vi "ScanAction.vi"(8 "error in (no error)":errorcluster caption="entrée d'erreur (pas d'erreur)", 9 "IndicePoint":i32, 10 "Dir":bool, 11 "Tools In":refnum<class "AttoAMC.lvclass"> caption="DNL_LabVIEW Object in") -> (0 "error out":errorcluster caption="sortie d'erreur", 2 "ScanParsOut":dbl[](array[numeric]), 3 "Tools Out":refnum<class "AttoAMC.lvclass"> caption="DNL_LabVIEW Object out")   [LabVIEW 2019, in "AttoAMC.lvclass"]
uses:
  AttoAMC.lvclass
  C:/Programmes Labview/LabScanV1A/DevicesClass/BaseDevice/BaseDevice.lvclass
  AttoAMC.lvclass/AttoAMC.ctl
  ScanActionStates.ctl
  <userlib>/GenProg/WritebyWeakRefNum.vi
  <vilib>/Utility/error.llb/Error Cluster From Error Code.vi
  <vilib>/ErrorRing/Error Ring.xnode
panel:
  in  "Reactivate":bool
  out "axis":u8
  out "Bkwd":bool
  out "Fwd":bool
  out "Trgt Rng(nm)":dbl
  in  "CtrlLpReact":u32
  out "PosDiff(nm)":dbl
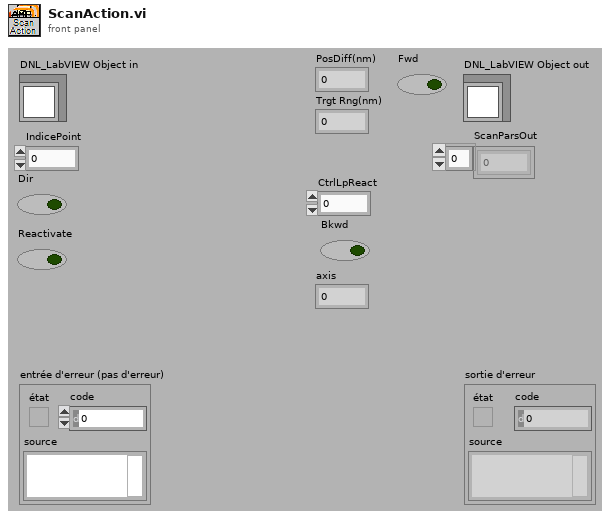
[diagram p1: front panel]
types:
  T1 = typedef "ScanActionStates.ctl" = enum16{"ReadPosDiff", "SetTarget", "WaitMoveDone", "MoveDone", "Timeout", "Ctrl_Loop_React", "Limit_check", "Error"}
  T2 = typedef "AttoAMC.lvclass/AttoAMC_Func.ctl" = enum16{"Position (um)"}
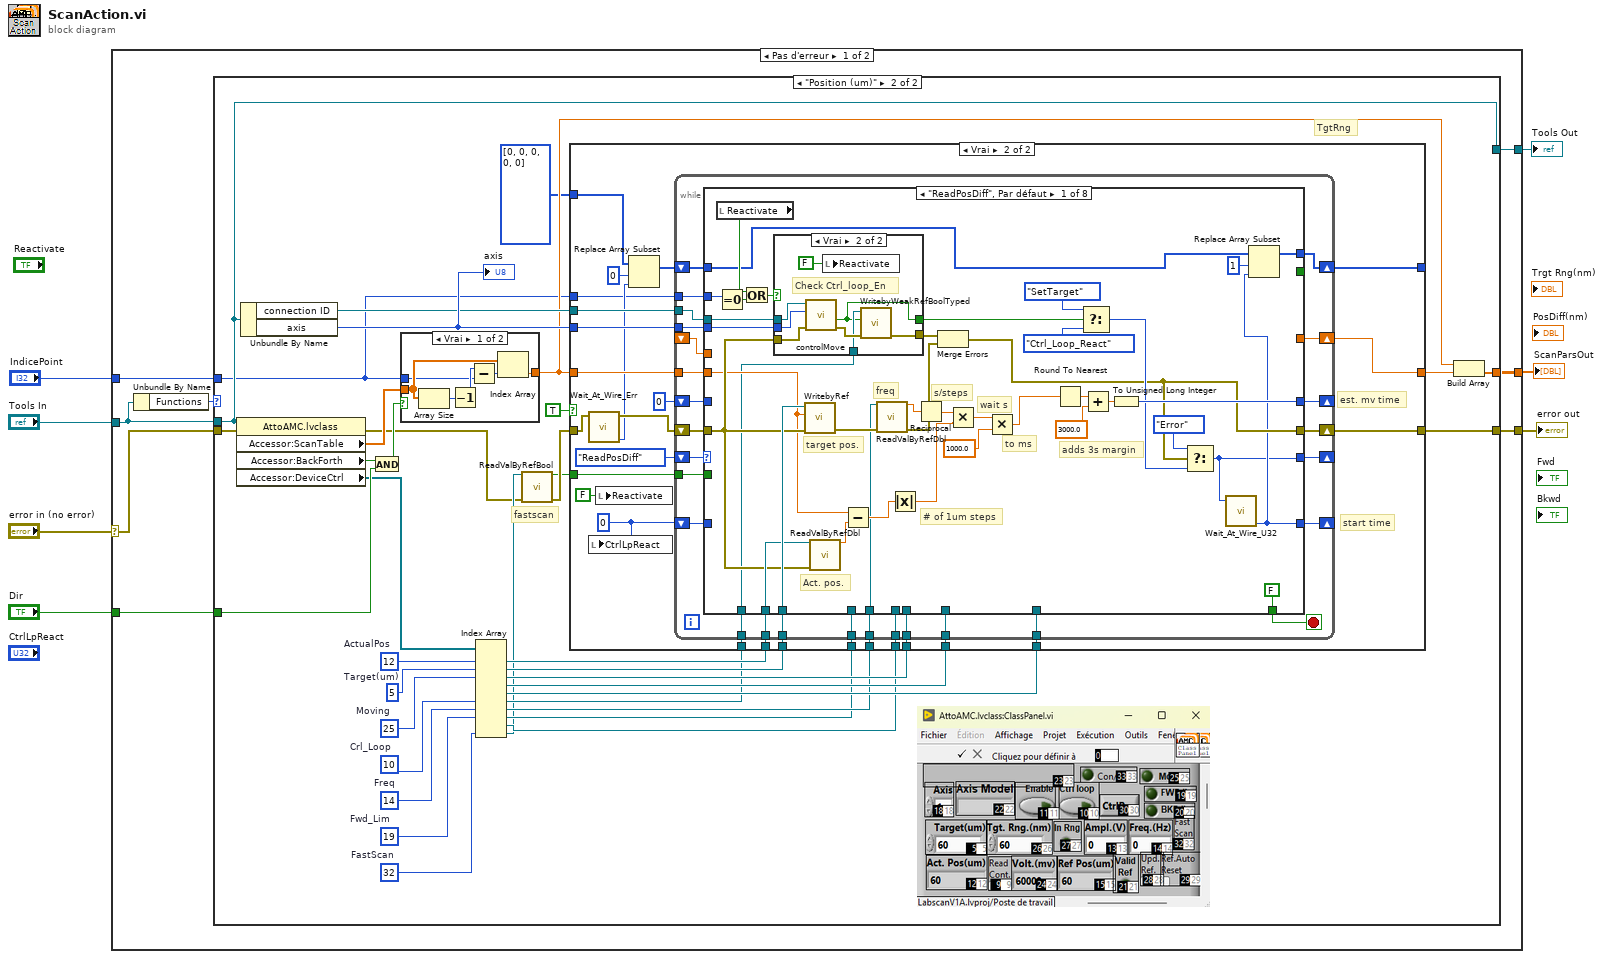
[diagram p0: block diagram]
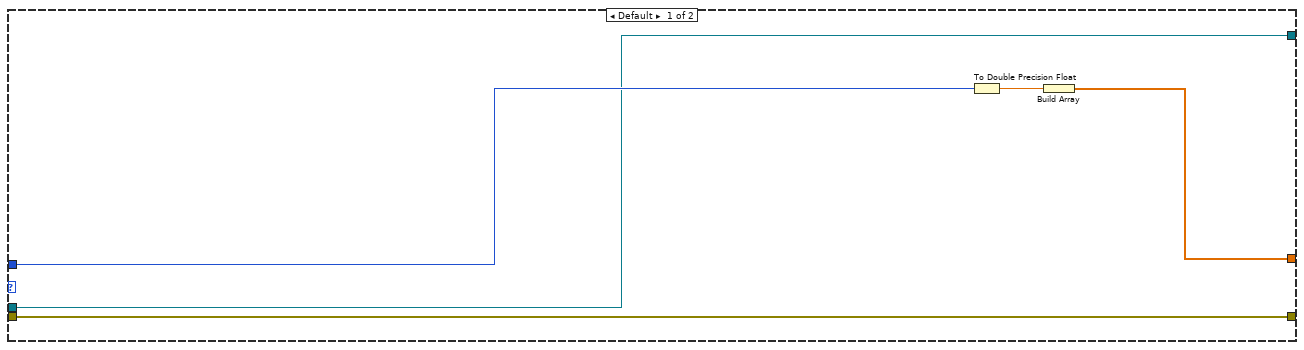
[diagram p2: hidden frame]
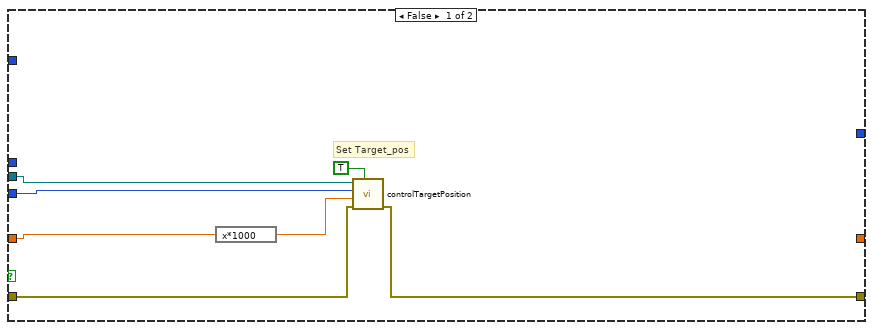
[diagram p3: hidden frame]
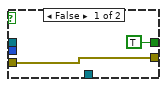
[diagram p4: hidden frame]
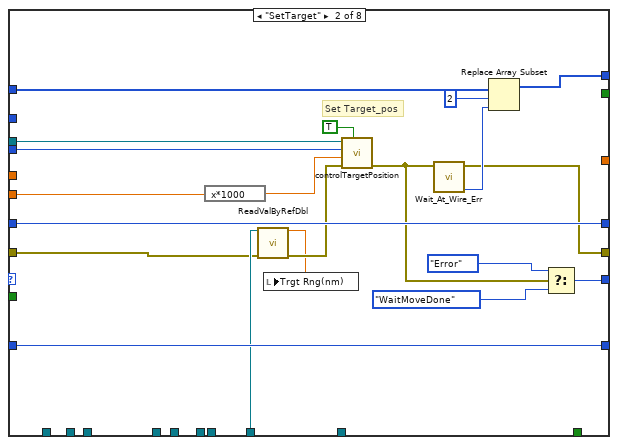
[diagram p5: hidden frame]
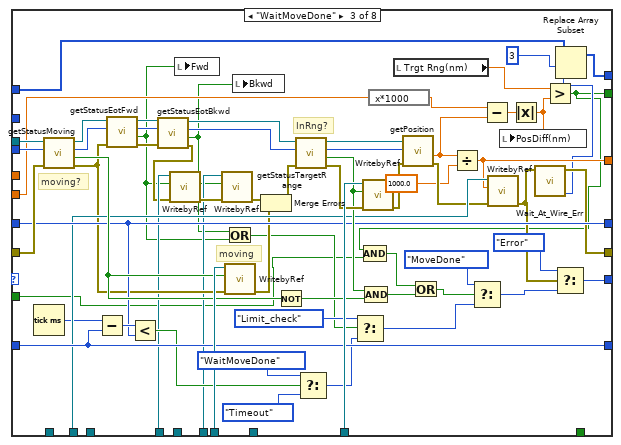
[diagram p6: hidden frame]
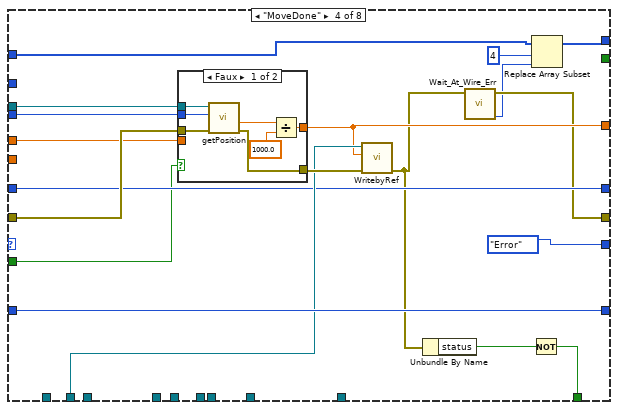
[diagram p7: hidden frame]
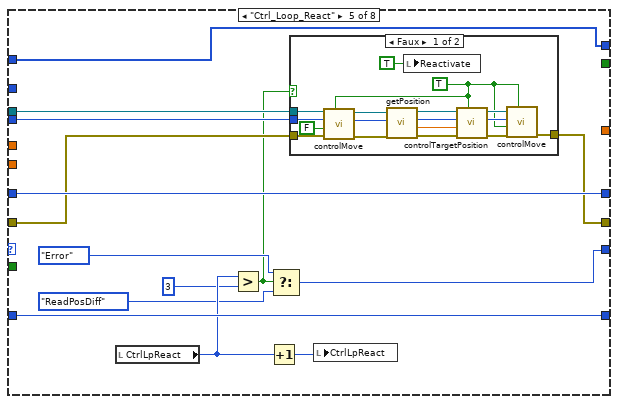
[diagram p9: hidden frame]
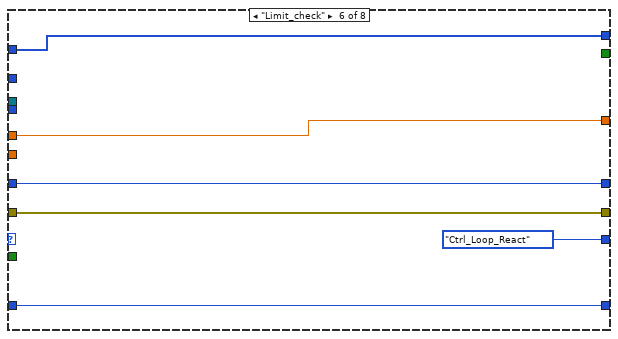
[diagram p11: hidden frame]
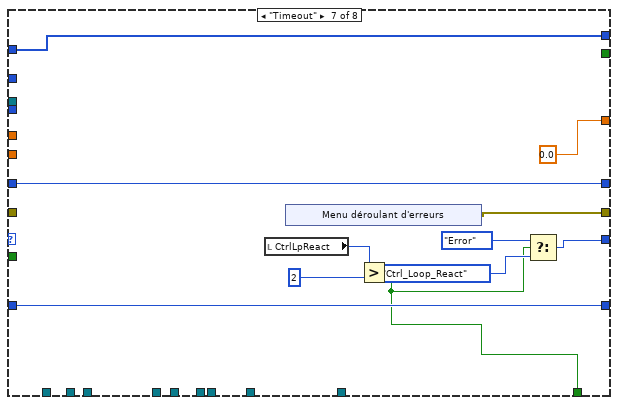
[diagram p12: hidden frame]
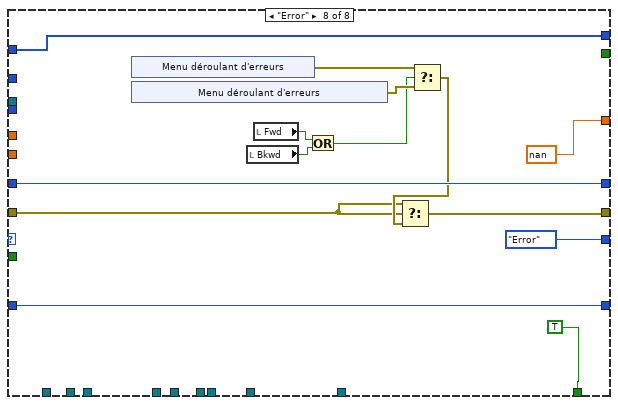
[diagram p13: hidden frame]
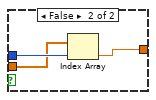
[diagram p14: hidden frame]
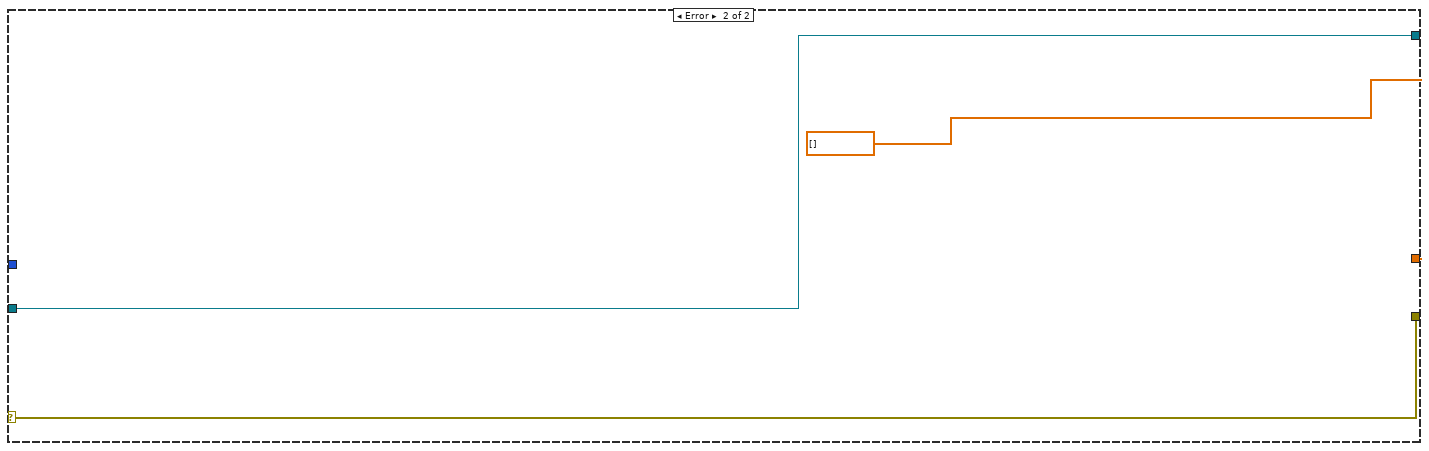
[diagram p15: hidden frame]
diagram:
  n1 = case shown="Pas d'erreur" "error in (no error)" {
    selector: "error in (no error)" -> [w12 w369]
    tunnel: "Tools In" -> [w13 w368]
    tunnel: [w11 dbl[] []] -> w2
    tunnel: [w10 w369] -> w5
    tunnel: [w9 w368] -> w4
    tunnel: "IndicePoint" -> [w14 _]
    tunnel: "Dir" -> [w8 _]
    frame No Error {
      n2 = Unbundle By Name(w13) -> ("Functions"=w15:T2)
      n3 = case shown="\"Position (um)\"" w15 {
        tunnel: [w16 w56] -> w11
        tunnel: w14 -> [w20 w21]
        tunnel: [w18 w55] -> w9
        tunnel: w13 -> [w18 w55]
        tunnel: w12 -> [w17 w54]
        tunnel: [w17 w42] -> w10
        tunnel: w8 -> [_ w50]
        frame Default {
          n4 = To Double Precision Float(number=w20) -> (double precision float=w19:dbl)
          n5 = Build Array(w19) -> (w16:dbl[])
        }
        frame "Position (um)" {
          w26 = 32  # FastScan
          w32 = 19  # Fwd_Lim
          w34 = 14  # Freq
          w36 = 10  # Crl_Loop
          w44 = 5  # Target(um)
          w47 = 25  # Moving
          w48 = 12  # ActualPos
          # "fastscan"
          # "TgtRng"
          n6 = property class="AttoAMC.lvclass"(reference=w55, error in=w54) -> (error out=w24:errorcluster, "Accessor:ScanTable"=w53:dbl[], "Accessor:BackForth"=w52:bool, "Accessor:DeviceCtrl"=w49:refnum<vi>[])  [unwired: 1 out]
          n7 = Unbundle By Name(w55) -> ("connection ID"=w40:refnum<k5>, "axis"=w41:u8)
          "axis" <- w41
          n8 = And(x=w52, y=w50) -> (x .and. y?=w51:bool)
          n9 = case shown="Vrai" w51 {
            tunnel: w21 -> [w358 w366]
            tunnel: [w363 w364] -> w29
            tunnel: w53 -> [w362 w365]
            frame True {
              n10 = Array Size(array=w362) -> (size(s)=w361:i32)
              n11 = Decrement(x=w361) -> (x-1=w359:i32)
              n12 = Subtract(x=w359, y=w358) -> (x-y=w360:i32)
              n13 = Index Array(array=w362, index=w360) -> (element=w363:dbl)
            }
            frame False {
              n14 = Index Array(array=w365, index=w366) -> (element=w364:dbl)
            }
          }
          n15 = Index Array(array=w49, index #1=w48, index #2=w44, index #3=w47, index #6=w36, index #7=w34, index #8=w32, index #10=w26) -> (element #1=w39:refnum<vi>, element #2=w45:refnum<vi>, element #3=w46:refnum<vi>, element #4=w37:refnum<vi>, element #5=w38:refnum<vi>, element #6=w35:refnum<vi>, element #7=w33:refnum<vi>, element #8=w31:refnum<vi>, element #9=w30:refnum<vi>, element #10=w25:refnum<vi>)  [unwired: 3 in]
          n16 = call <userlib>:"ReadValByRefBool.vi"("Control Ref"=w25, "error in"=w24) -> ("Valeur"=w22:bool, "error out"=w23:errorcluster)  [unwired: 12 in]
          n17 = case shown="Vrai" TRUE {
            tunnel: w46 -> [_ w90]
            tunnel: w45 -> [_ w89]
            tunnel: [_ w88] -> w43
            tunnel: [w57 w87] -> w42
            tunnel: w41 -> [w60 w86]
            tunnel: w40 -> [w61 w85]
            tunnel: w23 -> [w58 w73]
            tunnel: w39 -> [_ w84]
            tunnel: w38 -> [_ w81]
            tunnel: w37 -> [_ w80]
            tunnel: w35 -> [_ w79]
            tunnel: w33 -> [_ w78]
            tunnel: w31 -> [_ w77]
            tunnel: w30 -> [_ w76]
            tunnel: w29 -> [w59 w75]
            tunnel: u32[] [0, 0, 0, 0, 0] ("Clock(ms)") -> [_ w70]
            tunnel: [_ w67] -> _
            tunnel: w22 -> [_ w66]
            tunnel: w21 -> [_ w65]
            frame False {
              # "Set Target_pos"
              n18 = expression code="x*1000"(w59) -> (w62:dbl)
              n19 = call <userlib>:"controlTargetPosition.vi"("Set"=TRUE, "error in"=w58, "Target Position in"=w62, "axis in"=w60, "connection ID"=w61) -> ("error out"=w57:errorcluster)  [unwired: 3 in, 3 out]
            }
            frame True {
              w74 = u32 0 ("millisecond timer value")
              # "est. mv time"
              # "start time"
              n20 = call <userlib>:"Wait_At_Wire_Err.vi"("error in (no error)"=w73) -> ("Clock(ms)"=w68:u32, "error out"=w72:errorcluster)  [unwired: 8 in, 1 out]
              n21 = local write "CtrlLpReact"(w74) -> ()
              n22 = local write "Reactivate"(FALSE ("Reactivate")) -> ()
              n23 = Replace Array Subset(array=w70, new element=w68, index=0 ("indice")) -> (w71:u32[])
              n24 = while {
                tunnel: w90 -> [w117]
                tunnel: w89 -> [w116]
                tunnel: w81 -> [w114]
                tunnel: w86 -> [w112]
                tunnel: w85 -> [w111]
                tunnel: w84 -> [w109]
                shift-right: [w113] -> w87
                shift-left: w72 -> [w110]
                shift-right: [w106] -> _
                shift-left: w74 -> [w103]
                shift-right: [w105] -> _
                shift-left: ScanActionStates."ReadPosDiff" -> [w107]
                shift-right: [w102] -> _
                shift-left: u32 0 -> [w101]
                tunnel: w80 -> [w100]
                tunnel: w79 -> [w99]
                tunnel: w78 -> [w98]
                tunnel: w77 -> [w97]
                tunnel: w76 -> [w96]
                tunnel: w75 -> [w108]
                shift-right: [w95] -> w67
                shift-left: w71 -> [w94]
                tunnel: w66 -> [w93]
                tunnel: w65 -> [w92]
                shift-right: [w115] -> w88
                shift-left: _ -> [w91]
                stop <- w104 stop-if-true
                n25 = case shown="\"ReadPosDiff\", Par défaut" w107 {
                  tunnel: w117 -> [_ _ w251 _ _ _ _ _]
                  tunnel: w116 -> [w156 _ _ _ _ _ _ _]
                  tunnel: [_ _ w205 w264 _ w312 0.0 ("ScanParamIn") nan ("ScanParamIn")] -> w115
                  tunnel: w114 -> [_ _ w250 _ _ _ _ _]
                  tunnel: [w135 w167 w193 w258 w282 w315 w325 w335] -> w113
                  tunnel: w112 -> [w143 w177 w246 w266 w290 _ _ _]
                  tunnel: w111 -> [w144 w178 w247 w267 w291 _ _ _]
                  tunnel: w110 -> [w142 w179 w245 w265 w289 w315 _ w336]
                  tunnel: w109 -> [w152 _ w231 w268 _ _ _ _]
                  tunnel: w108 -> [w134 w175 w204 _ _ _ _ _]
                  tunnel: [w122 w183 w244 w269 w292 w316 w328 w345] -> w106
                  tunnel: [w121 w184 w235 ScanActionStates."Error" w283 ScanActionStates."Ctrl_Loop_React" w319 ScanActionStates."Error"] -> w105
                  tunnel: [FALSE _ _ w261 _ _ w320 TRUE] -> w104
                  tunnel: w103 -> [_ w183 w244 w269 w292 w316 w328 w345]
                  tunnel: [w148 w182 w241 w263 w293 w317 w327 w344] -> w102
                  tunnel: w101 -> [_ w182 w241 w263 w293 w317 w327 w344]
                  tunnel: w100 -> [_ w180 _ _ _ _ _ _]
                  tunnel: [_ _ w188 _ _ _ _ _] -> _
                  tunnel: w99 -> [w125 _ _ _ _ _ _ _]
                  tunnel: w98 -> [w146 _ _ _ _ _ _ _]
                  tunnel: w97 -> [_ _ w219 _ _ _ _ _]
                  tunnel: w96 -> [_ _ w218 _ _ _ _ _]
                  tunnel: [w127 w170 w197 w254 w280 w313 w318 w334] -> w95
                  tunnel: w94 -> [w118 w171 w196 w255 w280 w313 w318 w334]
                  tunnel: w93 -> [_ _ w189 w252 _ _ _ _]
                  tunnel: w92 -> [w124 _ _ _ _ _ _ _]
                  tunnel: w91 -> [_ _ _ w253 _ w312 _ _]
                  frame "ReadPosDiff", Default {
                    # "adds 3s margin"
                    # "to ms"
                    # "freq"
                    # "s/steps"
                    # "wait s"
                    # "# of 1um steps"
                    # "Act. pos."
                    # "target pos."
                    n26 = local read "Reactivate"() -> (w119:bool)
                    n27 = Equal To 0?(x=w124) -> (x = 0?=w123:bool)
                    n28 = Or(x=w119, y=w123) -> (x .or. y?=w120:bool)
                    n29 = case shown="Vrai" w120 {
                      tunnel: w144 -> [_ w166]
                      tunnel: w143 -> [_ w165]
                      tunnel: w142 -> [w158 w160]
                      tunnel: [w158 w163] -> w140
                      tunnel: [TRUE ("controll move out") w161] -> w136
                      tunnel: w125 -> [_ w162]
                      frame False {
                      }
                      frame True {
                        # "Check Ctrl_loop_En"
                        n30 = call <userlib>:"controlMove.vi"("error in"=w160, "axis in"=w165, "connection ID"=w166) -> ("error out"=w164:errorcluster, "controll move out"=w161:bool)  [unwired: 5 in, 2 out]
                        n31 = local write "Reactivate"(FALSE ("Reactivate")) -> ()
                        n32 = call <userlib>:"WritebyWeakRefBoolTyped.vi"("error in"=w164, "Valeur"=w161, "Control Ref"=w162) -> ("error out"=w163:errorcluster)  [unwired: 8 in]
                      }
                    }
                    n33 = call-poly <userlib>:"WritebyRef.vi"("error in"=w142, "Valeur"=w134, "Control Ref"=w156) -> ("error out"=w147:errorcluster)  [unwired: 8 in]
                    n34 = call <userlib>:"ReadValByRefDbl.vi"("Control Ref"=w152, "error in"=w142) -> ("Valeur"=w155:dbl)  [unwired: 12 in, 1 out]
                    n35 = Subtract(x=w134, y=w155) -> (x-y=w154:dbl)
                    n36 = call <userlib>:"ReadValByRefDbl.vi"("Control Ref"=w146, "error in"=w147) -> ("Valeur"=w145:dbl, "error out"=w141:errorcluster)  [unwired: 12 in]
                    n37 = Absolute Value(x=w154) -> (abs(x)=w131:dbl)
                    n38 = Reciprocal(x=w145) -> (1/x=w153:dbl)
                    n39 = Merge Errors(w140, w141) -> (w135:errorcluster)
                    n40 = Multiply(x=w153, y=w131) -> (x*y=w130:dbl)
                    n41 = Multiply(x=w130, y=1000.0) -> (x*y=w129:dbl)
                    n42 = Round To Nearest(number=w129) -> (nearest integer value=w149:dbl)
                    n43 = Select(t=ScanActionStates."SetTarget", s=w136, f=ScanActionStates."Ctrl_Loop_React") -> (s? t:f=w139:T1)
                    n44 = Add(x=w149, y=3000.0) -> (x+y=w133:dbl)
                    n45 = To Unsigned Long Integer(number=w133) -> (unsigned 32bit integer=w148:u32)
                    n46 = Select(t=ScanActionStates."Error", s=w135, f=w139) -> (s? t:f=w121:T1)
                    n47 = call <userlib>:"Wait_At_Wire_U32.vi"("error in (no error)"=w121) -> ("Clock(ms)"=w122:u32)  [unwired: 8 in, 2 out]
                    n48 = Replace Array Subset(array=w118, new element=w122, index=1 ("indice")) -> (w127:u32[])
                  }
                  frame "SetTarget" {
                    # "Set Target_pos"
                    n49 = expression code="x*1000"(w175) -> (w174:dbl)
                    n50 = call <userlib>:"ReadValByRefDbl.vi"("Control Ref"=w180, "error in"=w179) -> ("Valeur"=w173:dbl, "error out"=w181:errorcluster)  [unwired: 12 in]
                    n51 = local write "Trgt Rng(nm)"(w173) -> ()
                    n52 = call <userlib>:"controlTargetPosition.vi"("Set"=TRUE, "error in"=w181, "Target Position in"=w174, "axis in"=w177, "connection ID"=w178) -> ("error out"=w172:errorcluster)  [unwired: 3 in, 3 out]
                    n53 = call <userlib>:"Wait_At_Wire_Err.vi"("error in (no error)"=w172) -> ("Clock(ms)"=w168:u32, "error out"=w167:errorcluster)  [unwired: 8 in, 1 out]
                    n54 = Replace Array Subset(array=w171, new element=w168, index=2 ("indice")) -> (w170:u32[])
                    n55 = Select(t=ScanActionStates."Error", s=w172, f=ScanActionStates."WaitMoveDone") -> (s? t:f=w184:T1)
                  }
                  frame "WaitMoveDone" {
                    # "moving"
                    # "InRng?"
                    # "moving?"
                    n56 = Tick Count (ms)() -> (millisecond timer value=w198:u32)
                    n57 = call <userlib>:"getStatusMoving.vi"("error in"=w245, "axis in"=w246, "connection ID"=w247) -> ("error out"=w221:errorcluster, "status moving out"=w248:bool, "axis out"=w225:u8, "connection ID"=w226:refnum<k5>)  [unwired: 5 in]
                    n58 = Subtract(x=w198, y=w244) -> (x-y=w242:u32)
                    n59 = call <userlib>:"getStatusEotFwd.vi"("error in"=w221, "axis in"=w225, "connection ID"=w226) -> ("error out"=w228:errorcluster, "Status EOT FWD out"=w199:bool, "axis out"=w227:u8, "connection ID"=w224:refnum<k5>)  [unwired: 5 in]
                    n60 = Less?(x=w242, y=w241) -> (x < y?=w238:bool)
                    n61 = call <userlib>:"getStatusEotBkwd.vi"("error in"=w228, "axis in"=w227, "connection ID"=w224) -> ("error out"=w217:errorcluster, "Get Stus EOT BKWD out"=w200:bool, "axis out"=w222:u8, "connection ID"=w223:refnum<k5>)  [unwired: 5 in]
                    n62 = call-poly <userlib>:"WritebyRef.vi"("error in"=w217, "Valeur"=w199, "Control Ref"=w219) -> ("error out"=w220:errorcluster)  [unwired: 8 in]
                    n63 = local write "Fwd"(w199) -> ()
                    n64 = call-poly <userlib>:"WritebyRef.vi"("error in"=w220, "Valeur"=w200, "Control Ref"=w218) -> ("error out"=w214:errorcluster)  [unwired: 8 in]
                    n65 = Or(x=w200, y=w199) -> (x .or. y?=w211:bool)
                    n66 = call-poly <userlib>:"WritebyRef.vi"("error in"=w221, "Valeur"=w248, "Control Ref"=w251) -> ("error out"=w216:errorcluster)  [unwired: 8 in]
                    n67 = local write "Bkwd"(w200) -> ()
                    n68 = Merge Errors(w214, w216) -> (w215:errorcluster)
                    n69 = Not(x=w248) -> (.not. x?=w213:bool)
                    n70 = call <userlib>:"getStatusTargetRange.vi"("error in"=w215, "axis in"=w222, "connection ID"=w223) -> ("error out"=w249:errorcluster, "Status Target Range out"=w243:bool, "axis out"=w233:u8, "connection ID"=w234:refnum<k5>)  [unwired: 5 in]
                    n71 = Select(t=ScanActionStates."WaitMoveDone", s=w238, f=ScanActionStates."Timeout") -> (s? t:f=w208:T1)
                    n72 = Select(t=ScanActionStates."Limit_check", s=w211, f=w208) -> (s? t:f=w209:T1)
                    n73 = call-poly <userlib>:"WritebyRef.vi"("error in"=w249, "Valeur"=w243, "Control Ref"=w250) -> ("error out"=w232:errorcluster)  [unwired: 8 in]
                    n74 = Compound Arithmetic op=AND(w243, w213) -> (w191:bool)
                    n75 = expression code="x*1000"(w204) -> (w203:dbl)
                    n76 = local read "Trgt Rng(nm)"() -> (w206:dbl)
                    n77 = call <userlib>:"getPosition.vi"("error in"=w232, "axis in"=w233, "connection ID"=w234) -> ("error out"=w202:errorcluster, "position out"=w207:dbl)  [unwired: 5 in, 2 out]
                    n78 = Divide(x=w207, y=1000.0 ("x")) -> (x/y=w205:dbl)
                    n79 = Subtract(x=w203, y=w207) -> (x-y=w230:dbl)
                    n80 = call-poly <userlib>:"WritebyRef.vi"("error in"=w202, "Valeur"=w205, "Control Ref"=w231) -> ("error out"=w194:errorcluster)  [unwired: 8 in]
                    n81 = Absolute Value(x=w230) -> (abs(x)=w229:dbl)
                    n82 = local write "PosDiff(nm)"(w229) -> ()
                    n83 = call <userlib>:"Wait_At_Wire_Err.vi"("error in (no error)"=w194) -> ("Clock(ms)"=w192:u32, "error out"=w193:errorcluster)  [unwired: 8 in, 1 out]
                    n84 = Greater?(x=w206, y=w229) -> (0:w188:bool)
                    n85 = Compound Arithmetic op=AND(w188, w189) -> (w187:bool)
                    n86 = Or(x=w187, y=w191) -> (x .or. y?=w190:bool)
                    n87 = Select(t=ScanActionStates."MoveDone", s=w190, f=w209) -> (s? t:f=w239:T1)
                    n88 = Select(t=ScanActionStates."Error", s=w194, f=w239) -> (s? t:f=w235:T1)
                    n89 = Replace Array Subset(array=w196, new element=w192, index=3 ("indice")) -> (w197:u32[])
                  }
                  frame "MoveDone" {
                    n90 = case shown="Faux" w252 {
                      tunnel: [w277 w279] -> w270
                      tunnel: w267 -> [w275 _]
                      tunnel: w266 -> [w274 _]
                      tunnel: w265 -> [w273 w279]
                      tunnel: [w272 w278] -> w264
                      tunnel: w253 -> [_ w278]
                      frame False {
                        n91 = call <userlib>:"getPosition.vi"("error in"=w273, "axis in"=w274, "connection ID"=w275) -> ("error out"=w277:errorcluster, "position out"=w276:dbl)  [unwired: 5 in, 2 out]
                        n92 = Divide(x=w276, y=1000.0) -> (x/y=w272:dbl)
                      }
                      frame True {
                      }
                    }
                    n93 = call-poly <userlib>:"WritebyRef.vi"("error in"=w270, "Valeur"=w264, "Control Ref"=w268) -> ("error out"=w259:errorcluster)  [unwired: 8 in]
                    n94 = Unbundle By Name(w259) -> ("status"=w262:bool)
                    n95 = call <userlib>:"Wait_At_Wire_Err.vi"("error in (no error)"=w259) -> ("Clock(ms)"=w257:u32, "error out"=w258:errorcluster)  [unwired: 8 in, 1 out]
                    n96 = Not(x=w262) -> (.not. x?=w261:bool)
                    n97 = Replace Array Subset(array=w255, new element=w257, index=4 ("indice")) -> (w254:u32[])
                  }
                  frame "Ctrl_Loop_React" {
                    n98 = local read "CtrlLpReact"() -> (w287:u32)
                    n99 = Greater?(x=w287, y=u32 3) -> (0:w281:bool)
                    n100 = Increment(x=w287) -> (x+1=w288:u32)
                    n101 = Select(t=ScanActionStates."Error", s=w281, f=ScanActionStates."ReadPosDiff") -> (s? t:f=w283:T1)
                    n102 = case shown="Faux" w281 {
                      tunnel: w291 -> [w302 _]
                      tunnel: w290 -> [w301 _]
                      tunnel: w289 -> [w300 w311]
                      tunnel: [w305 w311] -> w282
                      frame False {
                        w296 = TRUE ("Set")
                        n103 = call <userlib>:"controlMove.vi"("Set"=w296, "error in"=w300, "control move in"=FALSE, "axis in"=w301, "connection ID"=w302) -> ("error out"=w299:errorcluster, "axis out"=w297:u8, "connection ID"=w298:refnum<k5>)  [unwired: 3 in, 1 out]
                        n104 = call <userlib>:"getPosition.vi"("error in"=w299, "axis in"=w297, "connection ID"=w298) -> ("error out"=w307:errorcluster, "position out"=w308:dbl, "axis out"=w309:u8, "connection ID"=w310:refnum<k5>)  [unwired: 5 in]
                        n105 = local write "Reactivate"(TRUE ("Reactivate")) -> ()
                        n106 = call <userlib>:"controlTargetPosition.vi"("Set"=w296, "error in"=w307, "Target Position in"=w308, "axis in"=w309, "connection ID"=w310) -> ("error out"=w306:errorcluster, "axis out"=w303:u8, "connection ID"=w304:refnum<k5>)  [unwired: 3 in, 1 out]
                        n107 = call <userlib>:"controlMove.vi"("Set"=w296, "error in"=w306, "control move in"=w296, "axis in"=w303, "connection ID"=w304) -> ("error out"=w305:errorcluster)  [unwired: 3 in, 3 out]
                      }
                      frame True {
                      }
                    }
                    n108 = local write "CtrlLpReact"(w288) -> ()
                  }
                  frame "Limit_check" {
                  }
                  frame "Timeout" {
                    n109 = local read "CtrlLpReact"() -> (w321:u32)
                    n110 = xnode "Menu déroulant d'erreurs"() -> ("sortie d'erreur"=w325:errorcluster)
                    n111 = Greater?(x=w321, y=u32 2) -> (0:w320:bool)
                    n112 = Select(t=ScanActionStates."Error", s=w320, f=ScanActionStates."Ctrl_Loop_React") -> (s? t:f=w319:T1)
                  }
                  frame "Error" {
                    n113 = xnode "Menu déroulant d'erreurs"() -> ("sortie d'erreur"=w342:errorcluster)
                    n114 = xnode "Menu déroulant d'erreurs"() -> ("sortie d'erreur"=w341:errorcluster)
                    n115 = local read "Bkwd"() -> (w339:bool)
                    n116 = local read "Fwd"() -> (w340:bool)
                    n117 = Or(x=w340, y=w339) -> (x .or. y?=w338:bool)
                    n118 = Select(t=w342, s=w338, f=w341) -> (s? t:f=w337:errorcluster)
                    n119 = Select(t=w336, s=w336, f=w337) -> (s? t:f=w335:errorcluster)
                  }
                }
              }
            }
          }
          n120 = Build Array(w29, w43) -> (w56:dbl[])
        }
      }
    }
    frame Error {
    }
  }
  "error out" <- w5
  "Tools Out" <- w4
  "ScanParsOut" <- w2
